vi "Build Device Table.vi"(8 "error in (no error)":errorcluster, 11 "HAL Editor in":refnum<class "HAL Editor.lvclass">) -> (0 "error out":errorcluster, 2 "Device Table":string[][](array[string]), 3 "HAL Editor out":refnum<class "HAL Editor.lvclass">)   [LabVIEW 2012, in "HAL Config.lvlib" / "HAL Editor.lvclass"]
uses:
  HAL Editor.lvclass
  build/ppl/lv-hal.lvlibp/Device/Device.lvclass
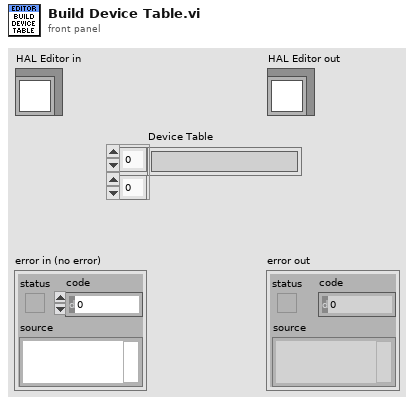
[diagram p1: front panel]
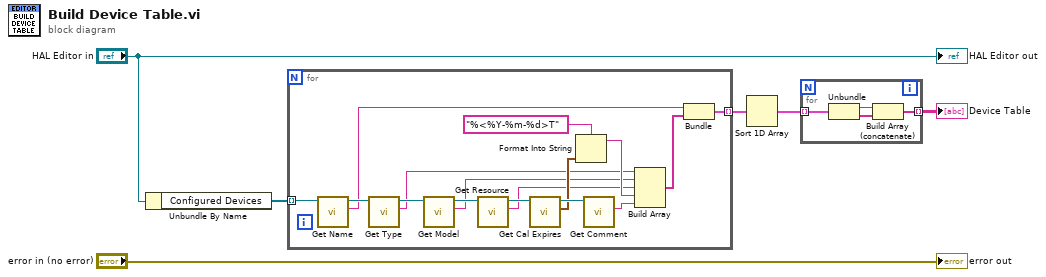
[diagram p0: block diagram]
diagram:
  n1 = Unbundle By Name("HAL Editor in") -> ("Configured Devices"=w4:refnum<class "Device.lvclass">[])
  n2 = for {
    tunnel: w4 -> [w22] mode=indexing
    tunnel: [w7] -> w3 mode=indexing
    n3 = call "Get Name.vi"("Device in"=w22) -> ("Name"=w8:string, "Device out"=w21:refnum<class "Device.lvclass">)  [unwired: 8 in, 1 out]
    n4 = call-dynamic "Get Type.vi"("Device in"=w21) -> ("Type"=w10:string, "Device out"=w20:refnum<class "Device.lvclass">)  [unwired: 8 in, 1 out]
    n5 = call-dynamic "Get Model.vi"("Device in"=w20) -> ("Model"=w11:string, "Device out"=w19:refnum<class "Device.lvclass">)  [unwired: 8 in, 1 out]
    n6 = call-dynamic "Get Resource.vi"("Device in"=w19) -> ("Resource"=w12:string, "Device out"=w18:refnum<class "Device.lvclass">)  [unwired: 8 in, 1 out]
    n7 = call "Get Cal Expires.vi"("Device in"=w18) -> ("Cal Expires"=w16:timestamp, "Device out"=w17:refnum<class "Device.lvclass">)  [unwired: 8 in, 1 out]
    n8 = Format Into String(format string="%<%Y-%m-%d>T", w16) -> (resulting string=w13:string)  [unwired: 2 in, 1 out]
    n9 = call "Get Comment.vi"("Device in"=w17) -> ("Comment"=w14:string)  [unwired: 8 in, 2 out]
    n10 = Build Array(w10, w11, w12, w13, w14) -> (w9:string[])
    n11 = Bundle("Name"=w8, w9) -> (w7:cluster{"Name":string, string[]})  [unwired: 1 in]
  }
  n12 = Sort 1D Array(array=w3) -> (sorted array=w2:cluster{"Name":string, string[]}[])
  n13 = for {
    tunnel: w2 -> [w26] mode=indexing
    tunnel: [w23] -> w1 mode=indexing
    n14 = Unbundle(w26) -> ("Name"=w25:string, w24:string[])
    n15 = Build Array (concatenate)(w25, w24) -> (w23:string[])
  }
  "Device Table" <- w1
  "error out" <- "error in (no error)"
  "HAL Editor out" <- "HAL Editor in"
